vi "MPVSenden.vi"(2 "Ventilposition":i32=1 min=1 max=6 step=1, 3 "FPGA VI Reference":refnum<k20>) -> (0 "Ventilposition":i32, 1 "FPGA VI Reference":refnum<k20>)   [LabVIEW 2010]
uses:
  <vilib>/rvi/interface/nirviMethod/nirviMethod.xnode
  C:/Users/HAGAR-IV/Desktop/Zeugs/markus/version feb 2012/FPGA Bitfiles/pertrasgcfpga2_FPGATarget_FPGA-Programm-10_16368CB6.lvbitx
  C:/Users/HAGAR-IV/Desktop/Zeugs/Johnny/pertrasgc fpga/FPGA-Programm-10-14.vi
  <vilib>/rvi/interface/common/niFpgaNodeNameForErrorReporting.ctl
  <vilib>/rvi/errors/niLvFpgaWhatHappensToTopLevelVI.ctl
  GVVentilposition.vi
  <vilib>/Utility/error.llb/Error Cluster From Error Code.vi
  <vilib>/rvi/errors/niLvFpgaAdjustHostInterfaceError.vi
  NiFpgaLv.dll
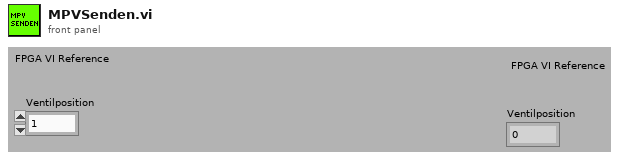
[diagram p1: front panel]
types:
  T1 = typedef "niFpgaNodeNameForErrorReporting.ctl" = enum16{"Open FPGA VI Reference", "Read/Write Control", "Invoke Method: Abort", "Invoke Method: Acknowledge IRQ", "Invoke Method: Download", "Invoke Method: FIFO.Configure", "Invoke Method: FIFO.Read", "Invoke Method: FIFO.Start", "Invoke Method: FIFO.Stop", "Invoke Method: FIFO.Write", "Invoke Method: Reset", "Invoke Method: Run", "Invoke Method: Wait on IRQ", "Close FPGA VI Reference"}
  T2 = typedef "niLvFpgaWhatHappensToTopLevelVI.ctl" = enum16{"top level VI scripted behind XNode", "top level VI inlined behind XNode"}
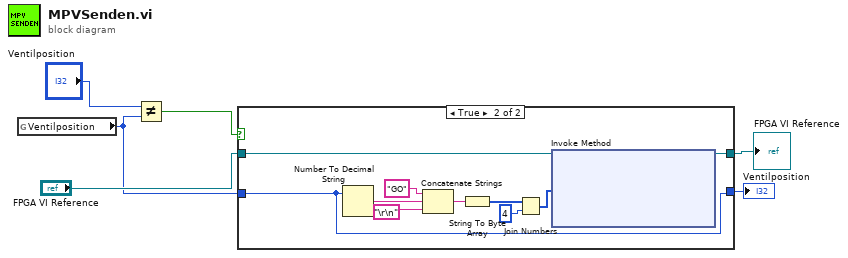
[diagram p0: block diagram]
diagram:
  n1 = global read "GVVentilposition.vi" "Ventilposition"() -> (w2:i32)
  n2 = Not Equal?(x="Ventilposition", y=w2) -> (x != y?=w3:bool)
  n3 = case shown="True" w3 {
    tunnel: "FPGA VI Reference" -> [w8 w18]
    tunnel: [w8 w10] -> w6
    tunnel: w2 -> [w7 w9]
    tunnel: [w7 w9] -> w1
    frame False {
    }
    frame True {
      n4 = Number To Decimal String(number=w9) -> (decimal integer string=w11:string)  [unwired: 1 in]
      n5 = Concatenate Strings("GO", w11, "\r\n") -> (w16:string)
      n6 = String To Byte Array(string=w16) -> (unsigned byte array=w15:u8[])
      n7 = Join Numbers(hi=w15, lo=u8 4) -> ((hi.lo)=w13:u16[])
      n8 = xnode "Invoke Method"("FPGA VI Reference In"=w18, "Data"=w13) -> ("FPGA VI Reference Out"=w10:refnum<k20>)  [unwired: 2 in, 2 out]
    }
  }
  "FPGA VI Reference" <- w6
  "Ventilposition" <- w1
